vi "CastArrayDependenciesToClusterOrClass.vi"(7 "Dependency Type (Class|Cluster)":variant, 8 "error in (no error)":errorcluster, 10 "index (-1: from start)":i32=-1, 11 "[Dependencies]":refnum<class>[](array[class])) -> (0 "error out":errorcluster, 3 "Dependencies output":variant)   [LabVIEW 2013, in "SMO.lvclass"]
uses:
  SMO.lvclass
  <vilib>/Utility/VariantDataType/VariantType.lvlib
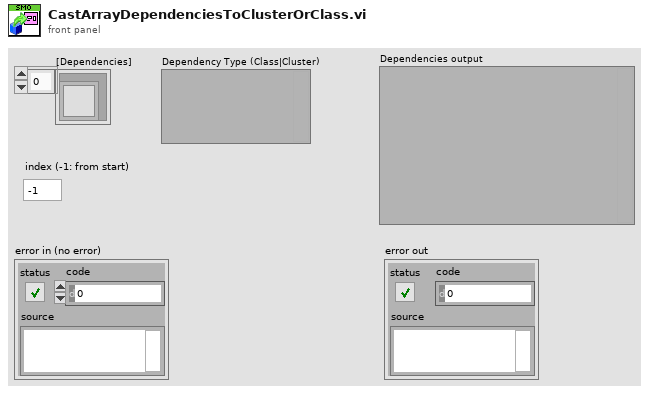
[diagram p1: front panel]
types:
  T1 = typedef "VariantType.lvlib/Type.ctl" = enum8{"Invalid Type", "Void", "I8", "I16", "I32", "I64", "U8", "U16", "U32", "U64", "Single Float", "Double Float", "Extended Float", "Single Complex", "Double Complex", "Extended Complex", "Enum U8", "Enum U16", "Enum U32", "Enum U64", "Single Float With Unit", "Double Float With Unit", "Extended Float With Unit", "Single Complex with Unit", "Double Complex with Unit", "Extended Complex with Unit", "Boolean", "String", "Path", "Picture", "Tag", "Array", "Cluster", "Variant", "LV Variant", "Waveform", "Timestamp", "Digital Waveform", "Digital Data", "ExpressData", "Refnum", "External Data", "VI", "Poly VI", "LabVIEW Class Instance", "Fixed Point"}
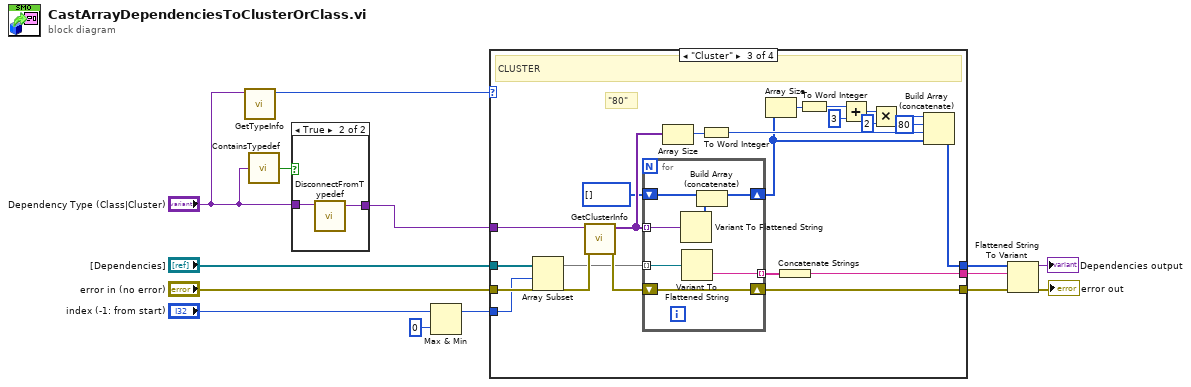
[diagram p0: block diagram]
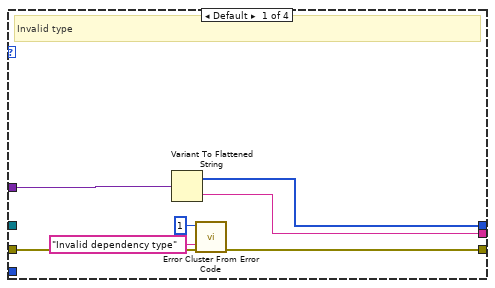
[diagram p3: hidden frame]
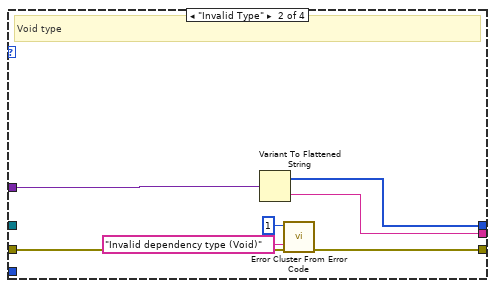
[diagram p4: hidden frame]
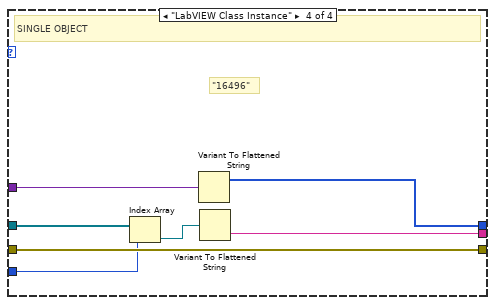
[diagram p5: hidden frame]
diagram:
  n1 = call <vilib>:"GetTypeInfo.vi"("Variant"="Dependency Type (Class|Cluster)") -> ("Type Enum"=w1:T1)  [unwired: 6 in, 4 out]
  n2 = call <vilib>:"ContainsTypedef.vi"("lvvar"="Dependency Type (Class|Cluster)") -> ("Contains Typedef"=w4:bool)
  n3 = case shown="True" w4 {
    tunnel: "Dependency Type (Class|Cluster)" -> [w15 w17]
    tunnel: [w15 w16] -> w3
    frame False {
    }
    frame True {
      n4 = call <vilib>:"DisconnectFromTypedef.vi"("lvvar in"=w17) -> ("lvvar out"=w16:variant)  [unwired: 4 in, 1 out]
    }
  }
  n5 = Max & Min(x="index (-1: from start)", y=0) -> (max(x,y)=w5:i32)  [unwired: 1 out]
  n6 = case shown="\"Cluster\"" w1 {
    tunnel: [w20 w27 w53 w66] -> w12
    tunnel: "[Dependencies]" -> [_ _ w34 w63]
    tunnel: "error in (no error)" -> [w21 w28 w52 w66]
    tunnel: [w22 w29 w45 w64] -> w9
    tunnel: [w23 w30 w37 w65] -> w8
    tunnel: w3 -> [w24 w31 w36 w67]
    tunnel: w5 -> [_ _ w32 w61]
    frame Default {
      # "Invalid type"
      n7 = Variant To Flattened String(Variant=w24) -> (data string=w22:string, 1:w23:i16[])
      n8 = call <vilib>:"Error Cluster From Error Code.vi"("error in (no error)"=w21, "error message (\"\")"="Invalid dependency type" ("error message (\"\")"), "error code (0)"=1) -> ("error out"=w20:errorcluster)  [unwired: 6 in]
    }
    frame "Invalid Type" {
      # "Void type"
      n9 = Variant To Flattened String(Variant=w31) -> (data string=w29:string, 1:w30:i16[])
      n10 = call <vilib>:"Error Cluster From Error Code.vi"("error in (no error)"=w28, "error message (\"\")"="Invalid dependency type (Void)" ("error message (\"\")"), "error code (0)"=1) -> ("error out"=w27:errorcluster)  [unwired: 6 in]
    }
    frame "Cluster" {
      # "\"80\""
      # "CLUSTER"
      n11 = Array Subset(array=w34, index=w32) -> (w33:refnum<class>[])  [unwired: 1 in]
      n12 = call <vilib>:"GetClusterInfo.vi"("error in (no error)"=w52, "Variant"=w36) -> ("error out"=w51:errorcluster, "Cluster Elements"=w50:variant[])  [unwired: 8 in]
      n13 = for {
        tunnel: w33 -> [w60] mode=indexing
        shift-right: [w59] -> w53
        shift-left: w51 -> [w59]
        tunnel: w50 -> [w58] mode=indexing
        shift-right: [w56] -> w38
        shift-left: i16[] [] -> [w57]
        tunnel: [w55] -> w46 mode=indexing
        n14 = Variant To Flattened String(Variant=w58) -> (1:w54:i16[])  [unwired: 1 out]
        n15 = Variant To Flattened String(Variant=w60) -> (data string=w55:string)  [unwired: 1 out]
        n16 = Build Array (concatenate)(w57, w54) -> (w56:i16[])
      }
      n17 = Array Size(array=w50) -> (size(s)=w49:i32)
      n18 = To Word Integer(number=w49) -> (16bit integer=w48:i16)
      n19 = Array Size(array=w38) -> (size(s)=w40:i32)
      n20 = Concatenate Strings(w46) -> (w45:string)
      n21 = To Word Integer(number=w40) -> (16bit integer=w44:i16)
      n22 = Add(x=w44, y=i16 3) -> (x+y=w42:i16)
      n23 = Multiply(x=w42, y=i16 2) -> (x*y=w39:i16)
      n24 = Build Array (concatenate)(w39, i16 80 ("16bit integer"), w48, w38) -> (w37:i16[])
    }
    frame "LabVIEW Class Instance" {
      # "\"16496\""
      # "SINGLE OBJECT"
      n25 = Index Array(array=w63, index=w61) -> (element=w62:refnum<class>)
      n26 = Variant To Flattened String(Variant=w67) -> (1:w65:i16[])  [unwired: 1 out]
      n27 = Variant To Flattened String(Variant=w62) -> (data string=w64:string)  [unwired: 1 out]
    }
  }
  n28 = Flattened String To Variant(4:w12, 6:w9, 7:w8) -> (0:→"error out":errorcluster, 3:→"Dependencies output":variant)
